vi "获得鉴权.vi"(8 "error in":errorcluster caption="错误输入（无错误）", 10 "Secret Key":string="rDKXbPRQq99dYX5rKlsBMlIGowxHm9mB", 11 "API Key":string="hWsGcQSG0ju0Z2SCZd4Pl32q") -> (0 "错误输出":errorcluster, 2 "access_token":string, 3 "client handle out":T1 caption="客户端句柄输出")   [LabVIEW 2025, in "Baidu api.lvlib"]
uses:
  Baidu api.lvlib
  <vilib>/httpClient/ClientHandle.ctl
  <vilib>/httpClient/POSTBuffer.vi
  <vilib>/httpClient/LabVIEWHTTPClient.lvlib
panel:
  out "body":string caption="体部"
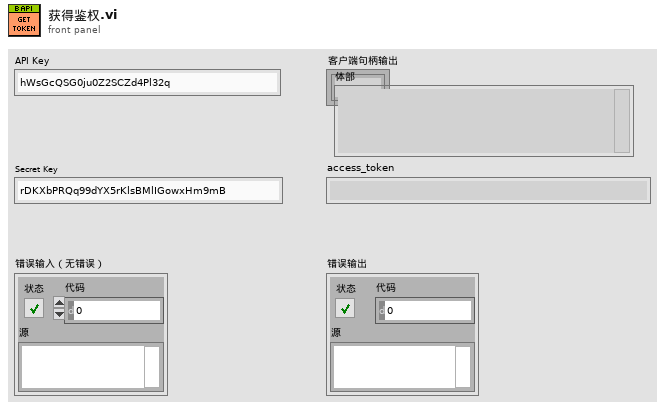
[diagram p1: front panel]
types:
  T1 = typedef "LabVIEWHTTPClient.lvlib/ClientHandle.ctl" = refnum<k1>
  T2 = cluster{"refresh_token":string, "expires_in":u64, "session_key":string, "access_token":string, "scope":string, "session_secret":string}
  T3 = cluster{"error":string, "error_description":string}
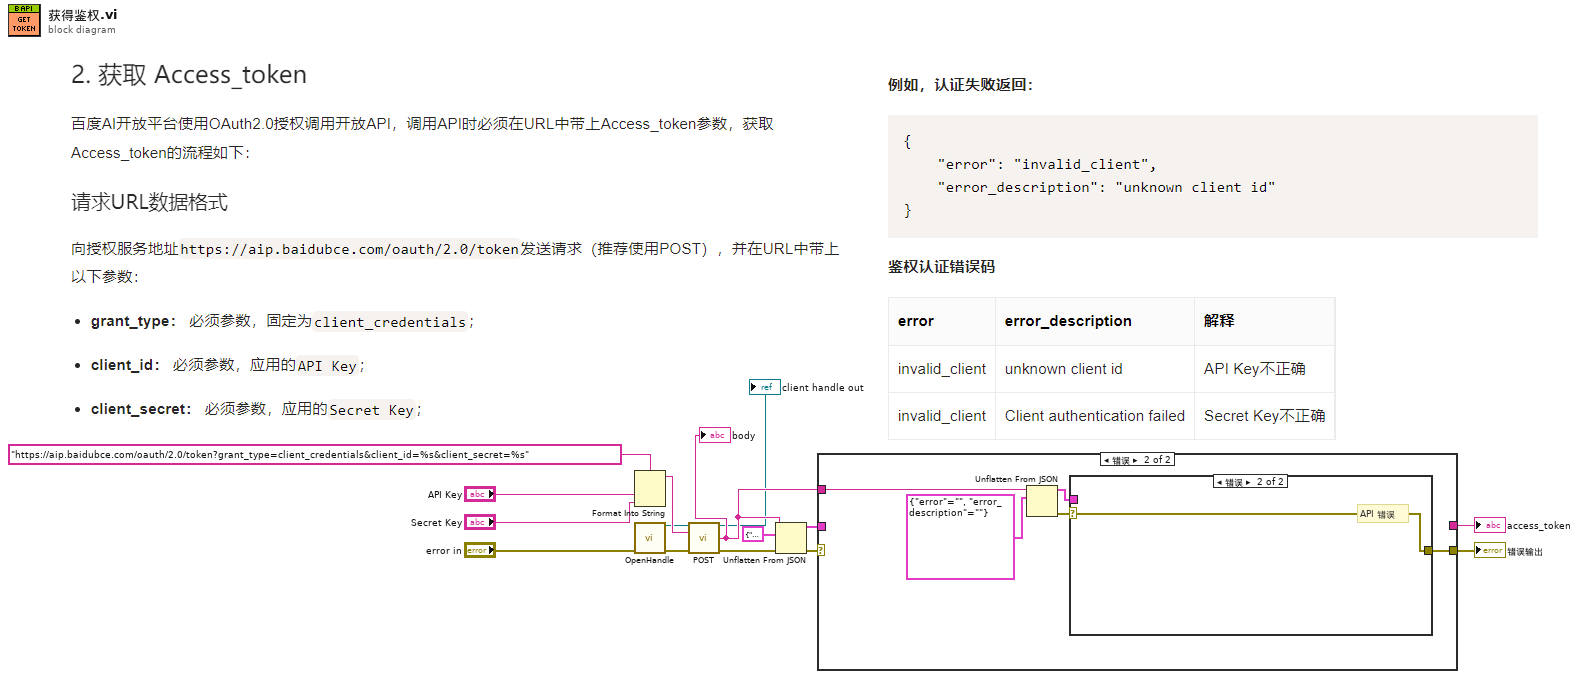
[diagram p0: block diagram]
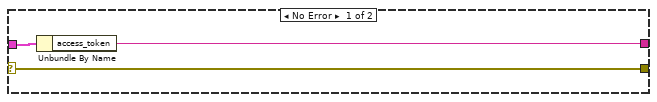
[diagram p2: hidden frame]
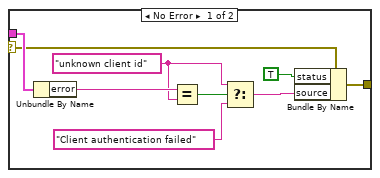
[diagram p3: hidden frame]
diagram:
  n1 = Format Into String(format string="https://aip.baidubce.com/oauth/2.0/token?grant_type=client_credentials&client_id=%s&client_secret=%s" ("url"), "API Key", "Secret Key") -> (resulting string=w11:string)  [unwired: 2 in, 1 out]
  n2 = call <vilib>:"OpenHandle.vi"("error in (no error)"="error in") -> ("client handle out"=w2:T1, "error out"=w12:errorcluster)  [unwired: 13 in]
  n3 = call-poly <vilib>:"POST.vi"("client handle"=w2, "url"=w11, "error in (no error)"=w12) -> ("client handle out"=→"client handle out":T1, "body"=w6:string, "error out"=w8:errorcluster)  [unwired: 9 in, 1 out]
  "body" <- w6
  n4 = Unflatten From JSON(JSON string=w6, type and defaults=T2 {"refresh_token"="", "expires_in"=0, "session_key"="", "access_token"="", "scope"="", "session_secret"=""} ("client_credentials"), error in (no error)=w8) -> (value=w5:T2, error out=w7:errorcluster)  [unwired: 4 in]
  n5 = case shown="错误" w7 {
    selector: w7 -> [w18 _]
    tunnel: w6 -> [_ w22]
    tunnel: [w18 w19] -> w3
    tunnel: w5 -> [w17 _]
    tunnel: [w16 _] -> w4
    frame No Error {
      n6 = Unbundle By Name(w17) -> ("access_token"=w16:string)
    }
    frame Error {
      n7 = Unflatten From JSON(JSON string=w22, type and defaults=T3 {"error"="", "error_description"=""}) -> (value=w21:T3, error out=w20:errorcluster)  [unwired: 5 in]
      n8 = case shown="错误" w20 {
        selector: w20 -> [w24 w33]
        tunnel: w21 -> [w32 _]
        tunnel: [w25 w33] -> w19
        frame No Error {
          w28 = "unknown client id" ("y")
          n9 = Unbundle By Name(w32) -> ("error"=w31:string)
          n10 = Equal?(x=w31, y=w28) -> (x = y?=w29:bool)
          n11 = Select(t=w28, s=w29, f="Client authentication failed" ("y")) -> (s? t:f=w26:string)
          n12 = Bundle By Name(cluster=w24, "status"=TRUE, "source"=w26) -> (w25:errorcluster)
        }
        frame Error {
          # "API 错误"
        }
      }
    }
  }
  "access_token" <- w4
  "错误输出" <- w3
